vi "ARC_Queue Lossy Enqueue.vi"(8 "error in (no error)":errorcluster caption="Error In (no error)", 9 "Data":variant, 10 "Event":string, 11 "Queue Name(unamed)":string) -> (0 "error out":errorcluster caption="Error Out", 1 "Overflow?":bool, 2 "Overflow Element":cluster{"Event":string, "Data":variant})   [LabVIEW 2016]
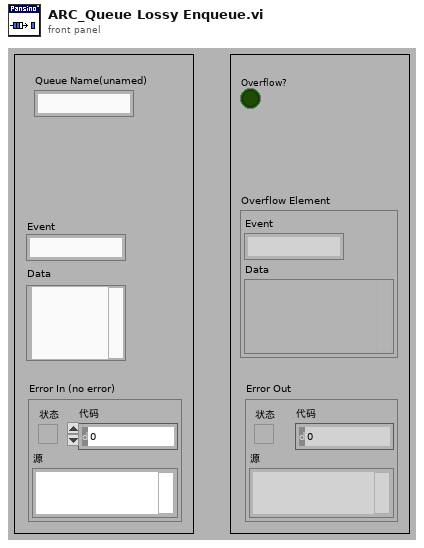
[diagram p1: front panel]
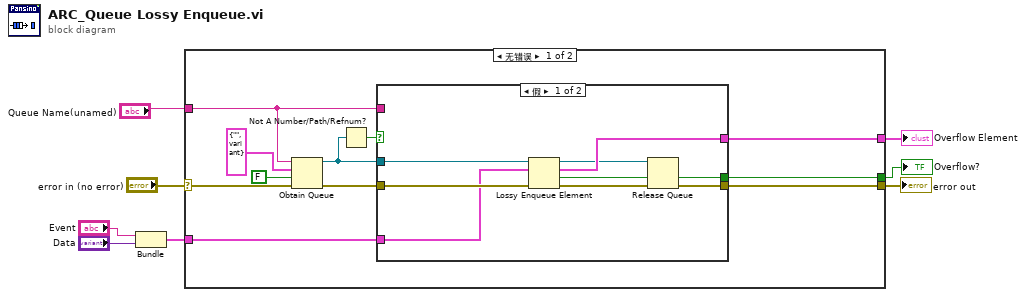
[diagram p0: block diagram]
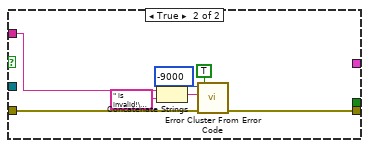
[diagram p2: hidden frame]
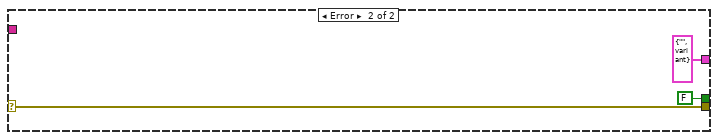
[diagram p3: hidden frame]
diagram:
  n1 = Bundle("Event"="Event", "Data"="Data") -> (w3:cluster{"Event":string, "Data":variant})  [unwired: 1 in]
  n2 = case shown="无错误" "error in (no error)" {
    selector: "error in (no error)" -> [w14 w37]
    tunnel: [w19 w37] -> w7
    tunnel: "Queue Name(unamed)" -> [w13 _]
    tunnel: w3 -> [w11 _]
    tunnel: [w10 FALSE ("overflow?")] -> w2
    tunnel: [w9 cluster{"Event":string, "Data":variant} {"Event"="", "Data"=variant} ("输出簇")] -> w1
    frame No Error {
      n3 = Obtain Queue(name (unnamed)=w13, element data type=cluster{"Event":string, "Data":variant} {"Event"="", "Data"=variant} ("输出簇"), create if not found? (T)=FALSE ("如未找到是否创建？(T)"), error in (no error)=w14) -> (queue out=w17:refnum<queue>, error out=w15:errorcluster)  [unwired: 1 in, 1 out]
      n4 = Not A Number/Path/Refnum?(number/path/refnum=w17) -> (NaN/Path/Refnum?=w16:bool)
      n5 = case shown="假" w16 {
        tunnel: w15 -> [w27 w30]
        tunnel: [w21 w29] -> w19
        tunnel: [w26 _] -> w9
        tunnel: [w25 _] -> w10
        tunnel: w13 -> [_ w28]
        tunnel: w17 -> [w24 _]
        tunnel: w11 -> [w20 _]
        frame False {
          n6 = Lossy Enqueue Element(queue=w24, element=w20, error in (no error)=w27) -> (queue out=w22:refnum<queue>, overflow element=w26:cluster{"Event":string, "Data":variant}, overflow?=w25:bool, error out=w23:errorcluster)
          n7 = Release Queue(queue=w22, error in (no error)=w23) -> (error out=w21:errorcluster)  [unwired: 1 in, 2 out]
        }
        frame True {
          n8 = Concatenate Strings(w28, " is invalid!\nEnsure the queue has been created!" ("字符串")) -> (w33:string)
          n9 = call <vilib>:"Error Cluster From Error Code.vi"("show call chain? (False)"=TRUE, "error in (no error)"=w30, "error message (\"\")"=w33, "error code (0)"=-9000) -> ("error out"=w29:errorcluster)  [unwired: 5 in]
        }
      }
    }
    frame Error {
    }
  }
  "error out" <- w7
  "Overflow?" <- w2
  "Overflow Element" <- w1
